vi "Write Timeout Interval.vi"(8 "error in (no error)":errorcluster, 10 "Timeout Interval (ms)":i32=-1, 11 "OnChange_Boolean in":refnum<class "OnChangeNotifier_Waveform.lvclass">) -> (0 "error out":errorcluster, 3 "OnChange_Boolean out":refnum<class "OnChangeNotifier_Waveform.lvclass">)   [LabVIEW 2021, in "OnChangeNotifier_Waveform.lvclass"]
uses:
  OnChangeNotifier_Waveform.lvclass
  OnChangeNotifier_Waveform.lvclass/OnChangeNotifier_Waveform.ctl
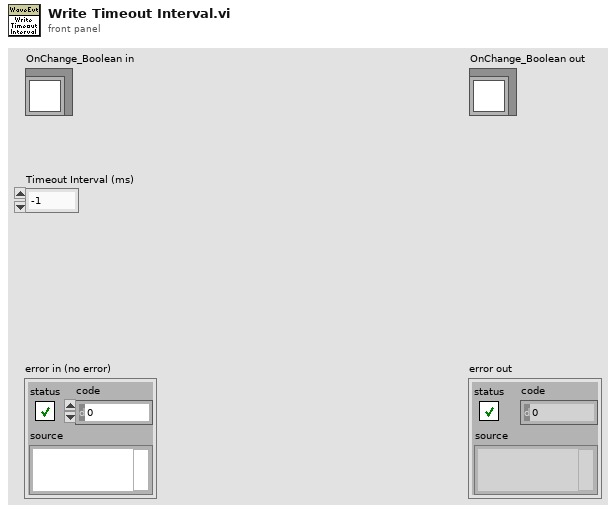
[diagram p1: front panel]
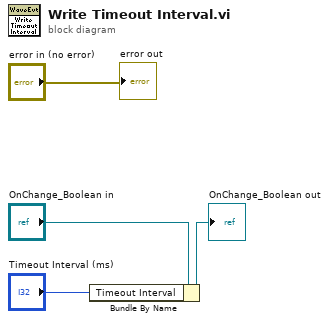
[diagram p0: block diagram]
diagram:
  n1 = Bundle By Name(cluster="OnChange_Boolean in", "Timeout Interval"="Timeout Interval (ms)") -> (→"OnChange_Boolean out":refnum<class "OnChangeNotifier_Waveform.lvclass">)
  "error out" <- "error in (no error)"
